vi "Discovery Client Register Service.vi"(5 "Request Data":T1={"service_description"={"display_name"="Dummy Test Service", "description_url"="", "provided_interfaces"=["UnitTestProvidedInterface"], "service_class"="UnitTestServiceClass", "attributes"=[]}, "location"={"location"="localhost", "insecure_port"="10001", "ssl_authenticated_port"=""}}, 11 "error in (no error)":errorcluster) -> (6 "Response Data":T4, 15 "error out":errorcluster)   [LabVIEW 2020]
uses:
  Discovery Client_lv/Discovery_client/RPC Messages/ni_measurementlink_discovery_v1_RegisterServiceResponse.ctl
  Discovery Client_lv/Discovery_client/RPC Messages/ni_measurementlink_discovery_v1_RegisterServiceRequest.ctl
  Discovery Client_lv/Discovery_client/RPC Messages/ni_measurementlink_discovery_v1_ServiceDescriptor.ctl
  Discovery Client_lv/Discovery_client/RPC Messages/ni_measurementlink_discovery_v1_ServiceLocation.ctl
  Discovery Client_lv/Discovery_client/Discovery_client.lvlib
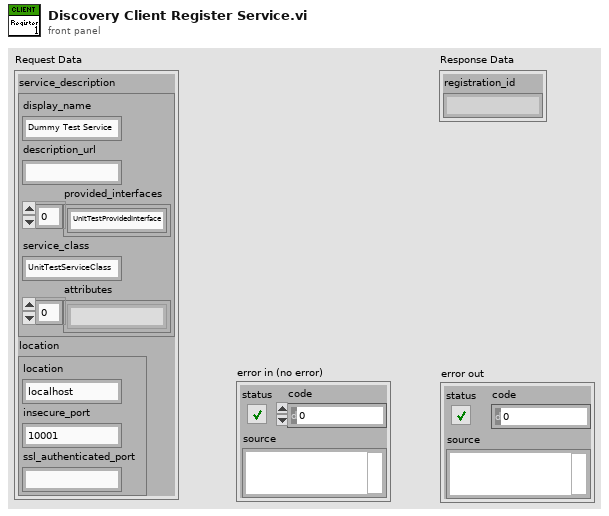
[diagram p1: front panel]
types:
  T1 = typedef "Discovery_client.lvlib/ni_measurementlink_discovery_v1_RegisterServiceRequest.ctl" = cluster{"service_description":T2, "location":T3}
  T2 = typedef "Discovery_client.lvlib/ni_measurementlink_discovery_v1_ServiceDescriptor.ctl" = cluster{"display_name":string, "description_url":string, "provided_interfaces":string[], "service_class":string, "attributes":string[]}
  T3 = typedef "Discovery_client.lvlib/ni_measurementlink_discovery_v1_ServiceLocation.ctl" = cluster{"location":string, "insecure_port":string, "ssl_authenticated_port":string}
  T4 = typedef "Discovery_client.lvlib/ni_measurementlink_discovery_v1_RegisterServiceResponse.ctl" = cluster{"registration_id":string}
  T5 = typedef "grpc-lvsupport-release.lvlib/grpcId.ctl" = u64
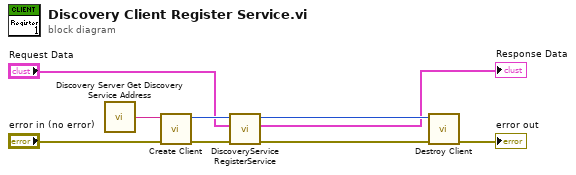
[diagram p0: block diagram]
diagram:
  n1 = call "Discovery Server Get Discovery Service Address.vi"() -> ("address"=w1:string)  [unwired: 15 in]
  n2 = call "Create Client.vi"("error in"="error in (no error)", "address"=w1) -> ("error out"=w7:errorcluster, "gRPC ID Out"=w9:T5)  [unwired: 8 in]
  n3 = call "DiscoveryService RegisterService.vi"("error in"=w7, "Request Data"="Request Data", "gRPC ID"=w9) -> ("error out"=w6:errorcluster, "Response Data"=→"Response Data":T4, "gRPC ID out"=w8:T5)  [unwired: 6 in]
  n4 = call "Destroy Client.vi"("error in"=w6, "gRPC ID"=w8) -> ("error out"=→"error out":errorcluster)  [unwired: 9 in]
